vi "Record UI Values.vi"(8 "error in (no error)":errorcluster, 9 "VI Ref":refnum<vi>, 10 "UI Dict":variant, 11 "PanelManager in":refnum<class "PanelManager.lvclass">) -> (0 "error out":errorcluster, 2 "UI Dict":variant, 3 "PanelManager out":refnum<class "PanelManager.lvclass">)   [LabVIEW 2015, in "PanelManager.lvclass"]
uses:
  PanelManager.lvclass
  <vilib>/Utility/traverseref.llb/TRef TravTarget.ctl
  <vilib>/Utility/traverseref.llb/VI Scripting - Traverse.lvlib
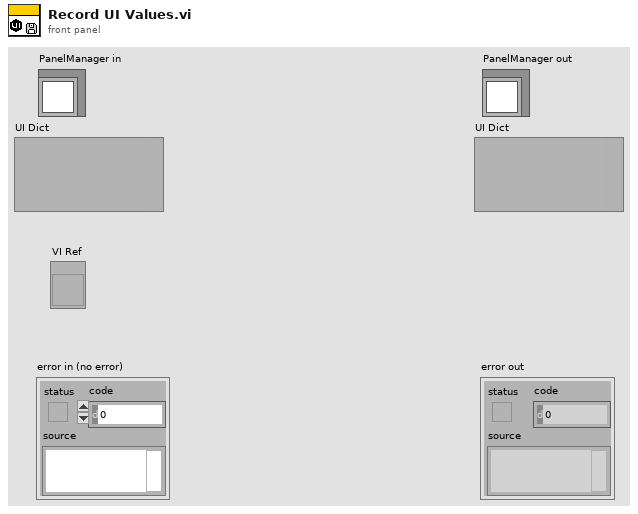
[diagram p1: front panel]
types:
  T1 = typedef "TRef TravTarget.ctl" = enum16{"FP", "BD", "Other"}
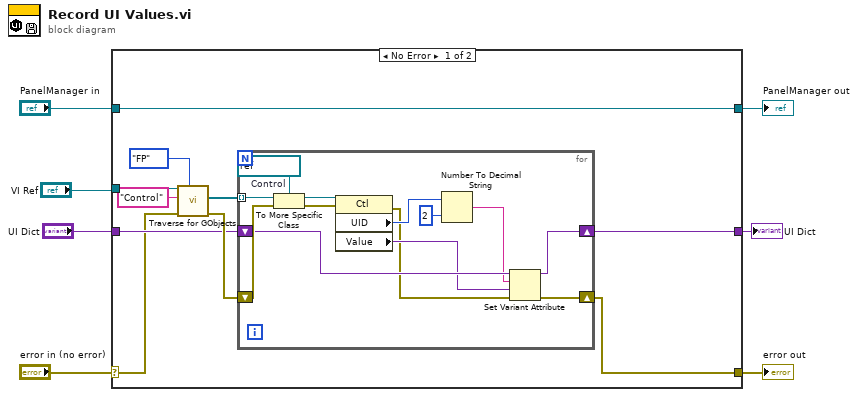
[diagram p0: block diagram]
diagram:
  n1 = case shown="No Error" "error in (no error)" {
    selector: "error in (no error)" -> [w10 w32]
    tunnel: [w9 w32] -> w6
    tunnel: [w17 w31] -> w4
    tunnel: "PanelManager in" -> [w17 w31]
    tunnel: "VI Ref" -> [w16 _]
    tunnel: "UI Dict" -> [w11 _]
    tunnel: [w8 _] -> w2
    frame No Error {
      n2 = call <vilib>:"Traverse for GObjects.vi"("Traverse Target"=TRef_TravTarget."FP", "error in (no error)"=w10, "Class Name"="Control", "VI Refnum"=w16) -> ("error out"=w12:errorcluster, "References"=w13:refnum<vi>[])  [unwired: 4 in, 2 out]
      n3 = for {
        tunnel: w13 -> [w30] mode=indexing
        shift-right: [w18] -> w8
        shift-left: w11 -> [w23]
        shift-right: [w19] -> w9
        shift-left: w12 -> [w29]
        w28 = refnum<vi> refnum  # Control
        n4 = To More Specific Class(target class=w28, reference=w30, error in=w29) -> (specific class reference=w27:refnum<vi>, error out=w26:errorcluster)
        n5 = property class="Ctl"(reference=w27, error in=w26) -> (error out=w20:errorcluster, "UID"=w25:i32, "Value"=w21:variant)  [unwired: 1 out]
        n6 = Number To Decimal String(number=w25, width (-)=i16 2) -> (decimal integer string=w22:string)
        n7 = Set Variant Attribute(Variant=w23, name=w22, value=w21, error in=w20) -> (Variant out=w18:variant, error out=w19:errorcluster)  [unwired: 1 out]
      }
    }
    frame Error {
    }
  }
  "error out" <- w6
  "PanelManager out" <- w4
  "UI Dict" <- w2
